vi "Format Path List.vi"(8 "Error in":errorcluster caption="Error in (no error)", 10 "Tree (F)":bool, 11 "Paths":path[](array[path])) -> (0 "Error out":errorcluster, 3 "Bullet List String":string)   [LabVIEW 2023, in "VIDoc Printer - Confluence.lvlib" / "VIDoc Printer - Confluence.lvclass"]
uses:
  VIDoc Printer - Confluence.lvclass
  VIDoc Printer - Confluence.lvclass/VIDoc Printer - Confluence.ctl
  Confluence Formatting/Confluence Formatting.lvlib
  Printer/VIDoc Printer.lvclass
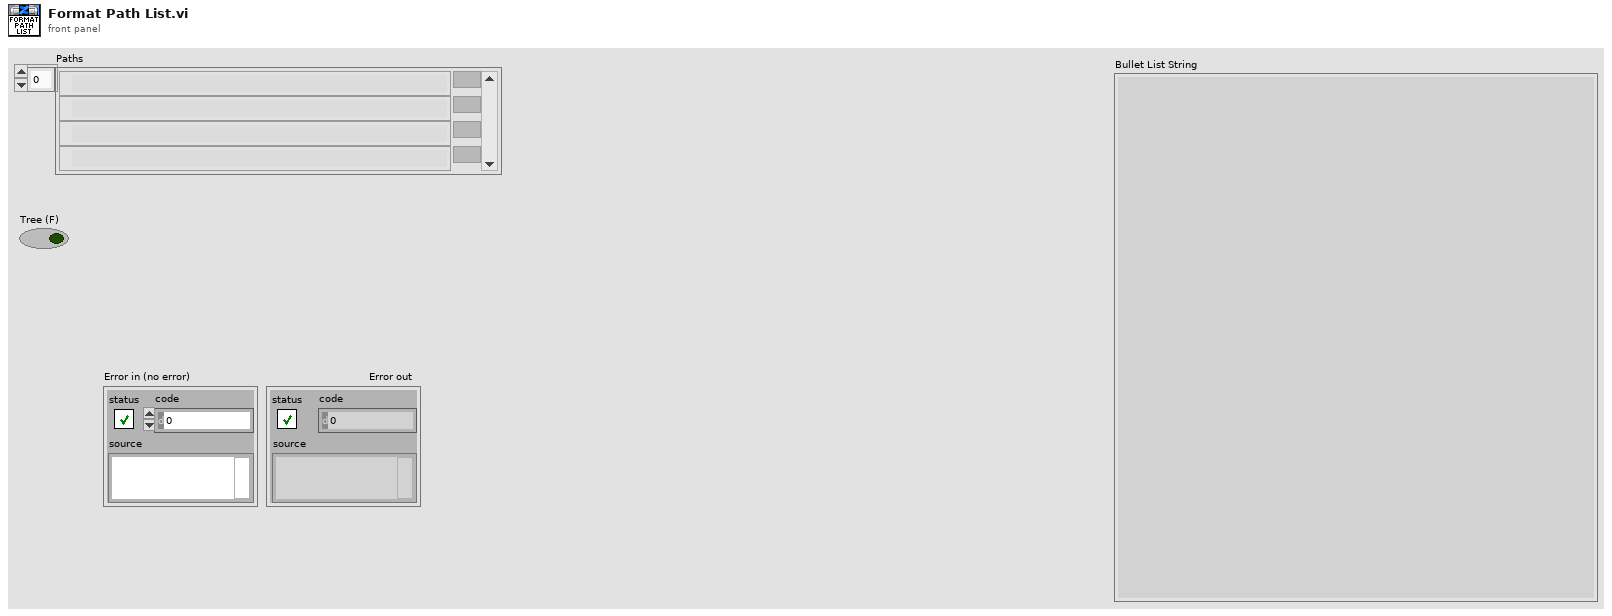
[diagram p1: front panel]
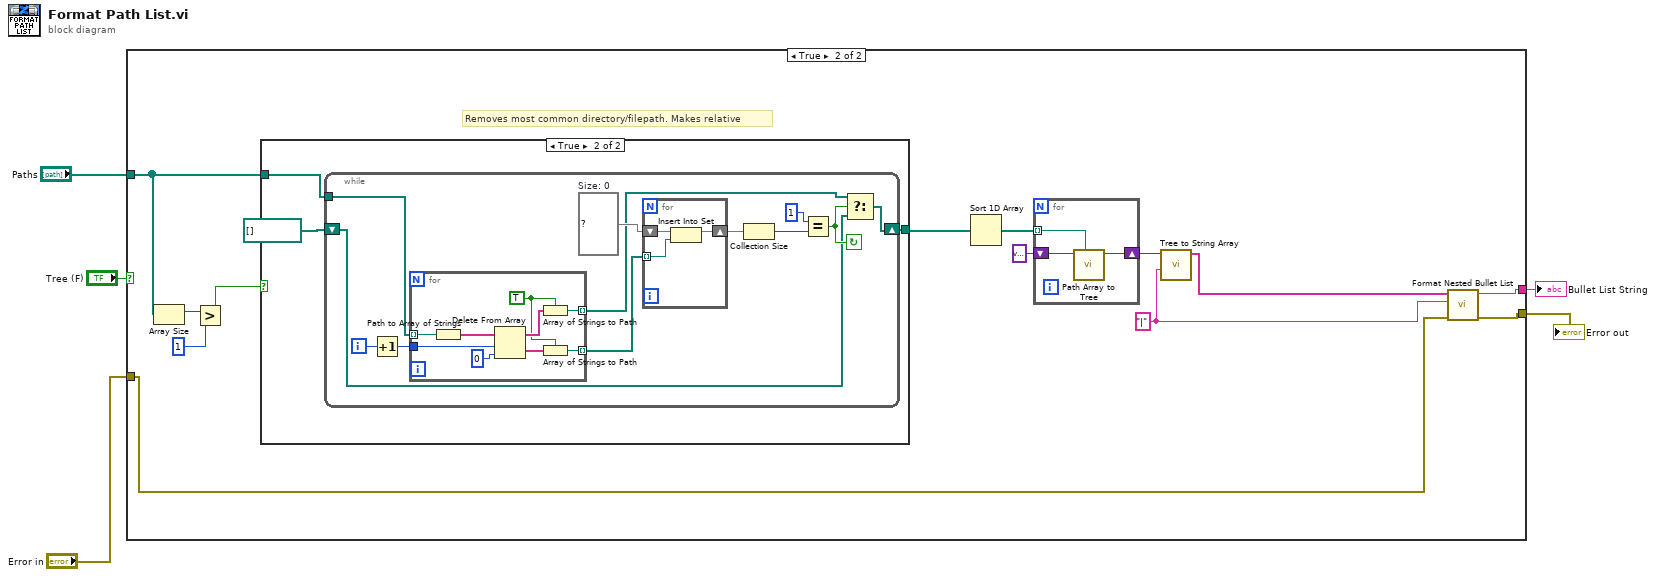
[diagram p0: block diagram]
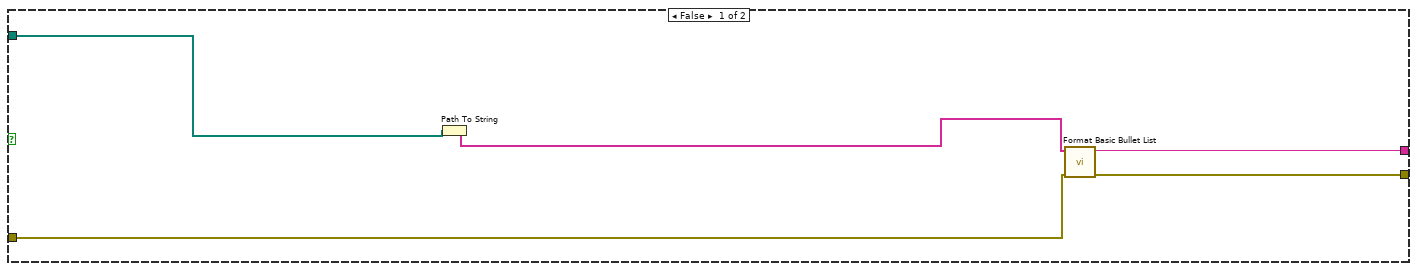
[diagram p2: hidden frame]
diagram:
  n1 = case shown="True" "Tree (F)" {
    tunnel: "Paths" -> [w10 w23]
    tunnel: [w9 w19] -> w1
    tunnel: "Error in" -> [w8 w17]
    tunnel: [w7 w18] -> w2
    frame False {
      n2 = Path To String(path=w10) -> (string=w6:string[])
      n3 = call "Format Basic Bullet List.vi"("Error in"=w8, "String Array"=w6) -> ("Error out"=w7:errorcluster, "Bullet List"=w9:string)  [unwired: 8 in]
    }
    frame True {
      w12 = "|"
      # "Removes most common directory/filepath. Makes relative"
      n4 = Array Size(array=w23) -> (size(s)=w22:i32)
      n5 = Greater?(x=w22, y=1) -> (0:w20:bool)
      n6 = case shown="True" w20 {
        tunnel: [w27 w30] -> w16
        tunnel: w23 -> [w27 w28]
        frame False {
        }
        frame True {
          n7 = while {
            tunnel: w28 -> [w42]
            shift-right: [w32] -> w30
            shift-left: path[] [] -> [w31]
            i -> [w41]
            stop <- w34 continue-if-true
            w38 = set{path} {}  # Size: 0
            n8 = Increment(x=w41) -> (x+1=w40:i32)
            n9 = for {
              tunnel: w42 -> [w54] mode=indexing
              tunnel: [w50] -> w39 mode=indexing
              tunnel: [w48] -> w33 mode=indexing
              tunnel: w40 -> [w47]
              w46 = TRUE ("relative")
              n10 = Path to Array of Strings(0:w54) -> (2:w53:string[])  [unwired: 1 out]
              n11 = Delete From Array(array=w53, length=w47, index=0) -> (deleted portion=w51:string[], array with subset deleted=w49:string[])
              n12 = Array of Strings to Path(0:w49, 1:w46) -> (2:w48:path)
              n13 = Array of Strings to Path(0:w51, 1:w46) -> (2:w50:path)
            }
            n14 = for {
              tunnel: w39 -> [w45] mode=indexing
              shift-right: [w44] -> w37
              shift-left: w38 -> [w43]
              n15 = Insert Into Set(10:w45, 11:w43) -> (3:w44:set{path})  [unwired: 1 out]
            }
            n16 = Collection Size(1:w37) -> (0:w36:i32)
            n17 = Equal?(x=1, y=w36) -> (x = y?=w34:bool)
            n18 = Select(t=w33, s=w34, f=w31) -> (s? t:f=w32:path[])
          }
        }
      }
      n19 = Sort 1D Array(array=w16) -> (sorted array=w15:path[])
      n20 = for {
        tunnel: w15 -> [w24] mode=indexing
        shift-right: [w25] -> w13
        shift-left: variant -> [w26]
        n21 = call "Path Array to Tree.vi"("Path"=w24, "Tree in"=w26) -> ("Tree out"=w25:variant)  [unwired: 9 in]
      }
      n22 = call "Tree to String Array.vi"("Delimiter (Tab)"=w12, "Tree in"=w13) -> ("String Array"=w11:string[])  [unwired: 9 in]
      n23 = call "Format Nested Bullet List.vi"("Error in"=w17, "Delimiter (Tab)"=w12, "String Array"=w11) -> ("Error out"=w18:errorcluster, "Nested Bullet List"=w19:string)  [unwired: 7 in]
    }
  }
  "Error out" <- w2
  "Bullet List String" <- w1
